vi "String to timestamp new.vi"(11 "String Timestamp":string) -> (3 "Timestamp":timestamp)   [LabVIEW 2017]
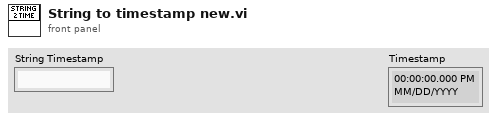
[diagram p1: front panel]
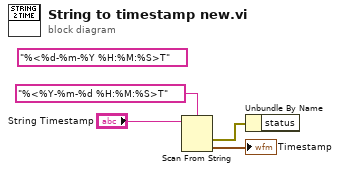
[diagram p0: block diagram]
diagram:
  (unwired) "%<%d-%m-%Y %H:%M:%S>T" ("format string")
  n1 = Scan From String(format string="%<%Y-%m-%d %H:%M:%S>T", input string="String Timestamp") -> (error out=w1:errorcluster, output 1=→"Timestamp":timestamp)  [unwired: 3 in, 2 out]
  n2 = Unbundle By Name(w1) -> ()  [unwired: 1 out]
